vi "initest.vi"() -> ()   [LabVIEW 2017]
uses:
  <vilib>/Utility/config.llb/Write Key (I32).vi
  <vilib>/Utility/config.llb/NI_LVConfig.lvlib
panel:
  out "error out":errorcluster
  in  "Error in":errorcluster
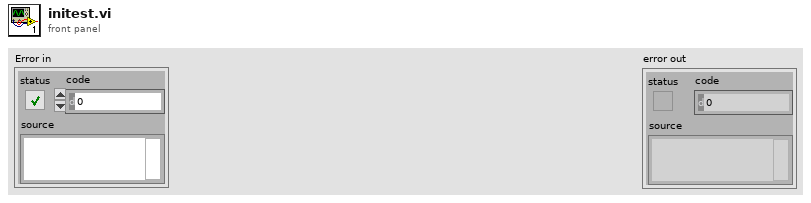
[diagram p1: front panel]
types:
  T1 = enum32{"invalid app kind", "Development System", "Run Time System", "Student Edition", "Embedded LabVIEW", "Evaluation", "Custom"}
  T2 = typedef "NI_LVConfig.lvlib/Config Data RefNum.ctl" = refnum<k1>
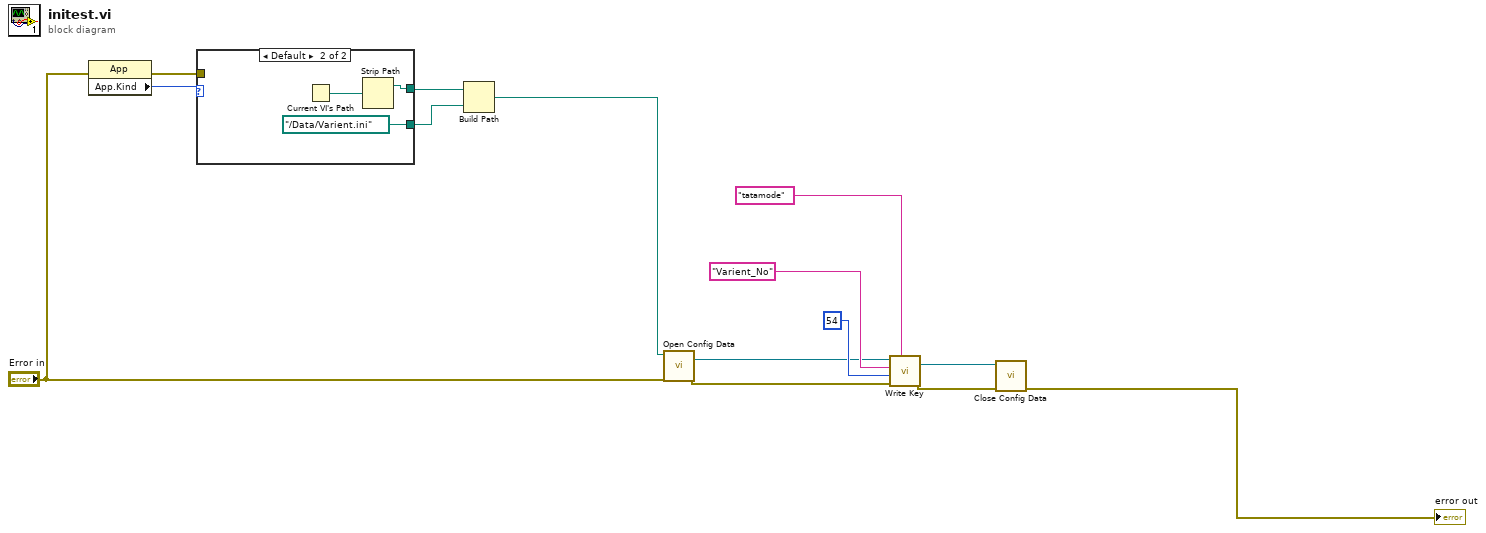
[diagram p0: block diagram]
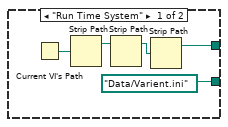
[diagram p2: hidden frame]
diagram:
  n1 = property class="App"(error in="Error in") -> (error out=w12:errorcluster, "App.Kind"=w14:T1)  [unwired: 1 in, 1 out]
  n2 = case shown="Default" w14 {
    tunnel: [path "Data/Varient.ini" ("path") path "../Data/Varient.ini" ("path")] -> w13
    tunnel: [w15 w20] -> w11
    tunnel: w12 -> [_ _]
    frame "Run Time System" {
      n3 = Current VI's Path() -> (path=w18:path)
      n4 = Strip Path(path=w18) -> (stripped path=w17:path)  [unwired: 1 out]
      n5 = Strip Path(path=w17) -> (stripped path=w16:path)  [unwired: 1 out]
      n6 = Strip Path(path=w16) -> (stripped path=w15:path)  [unwired: 1 out]
    }
    frame Default {
      n7 = Current VI's Path() -> (path=w21:path)
      n8 = Strip Path(path=w21) -> (stripped path=w20:path)  [unwired: 1 out]
    }
  }
  n9 = Build Path(base path=w11, name or relative path=w13) -> (appended path=w10:path)
  n10 = call <vilib>:"Open Config Data.vi"("error in (no error)"="Error in", "configuration file path"=w10) -> ("error out"=w4:errorcluster, "refnum"=w5:T2)  [unwired: 7 in, 1 out]
  n11 = call-poly <vilib>:"Write Key.vi"("section"="tatamode", "error in (no error)"=w4, "value"=54, "key"="Varient_No", "refnum"=w5) -> ("error out"=w2:errorcluster, "refnum out"=w3:T2)  [unwired: 4 in, 1 out]
  n12 = call <vilib>:"Close Config Data.vi"("error in (no error)"=w2, "refnum"=w3) -> ("error out"=→"error out":errorcluster)  [unwired: 8 in, 1 out]
